vi "AeroQuadUploader32 - Copy.vi"() -> ()   [LabVIEW 2010]
panel:
  in  "WebBrowser":refnum<k7>(container)
  in  "URL":string="http://aq32.aeroquad.com"
  in  "Com Port":refnum<visa-resource-name>
  out "Status":string="AeroQuad 32 Uploader"
  in  "Restart":bool
  in  "Done":bool
  in  "Upload":bool
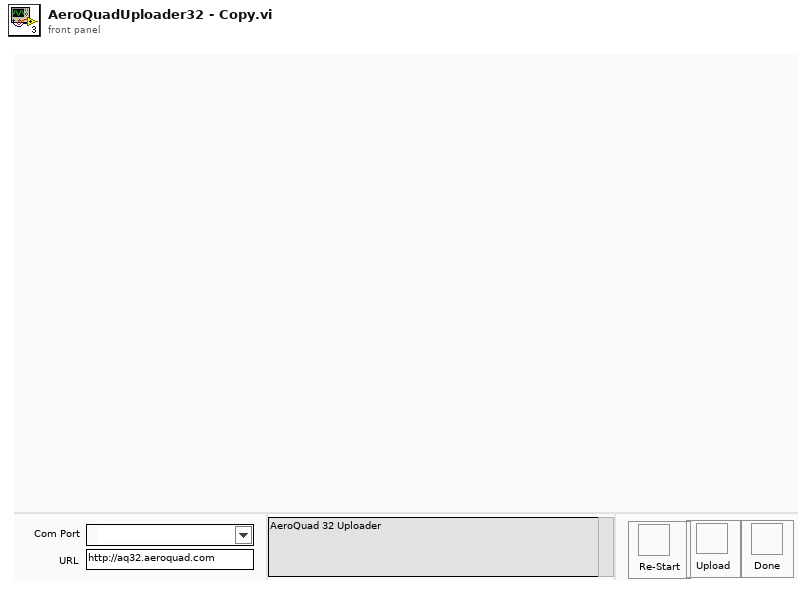
[diagram p1: front panel]
types:
  T1 = cluster{"Connected":bool, "WebBrowser":refnum<k7>, "WorkingFolder":path, "HTML":string}
  T2 = enum16{"Read", "Write", "ReadWrite", "BufferedRead", "BufferedReadWrite"}
  T3 = enum32{"invalid app kind", "Development System", "Run Time System", "Student Edition", "Embedded LabVIEW", "Evaluation", "Custom"}
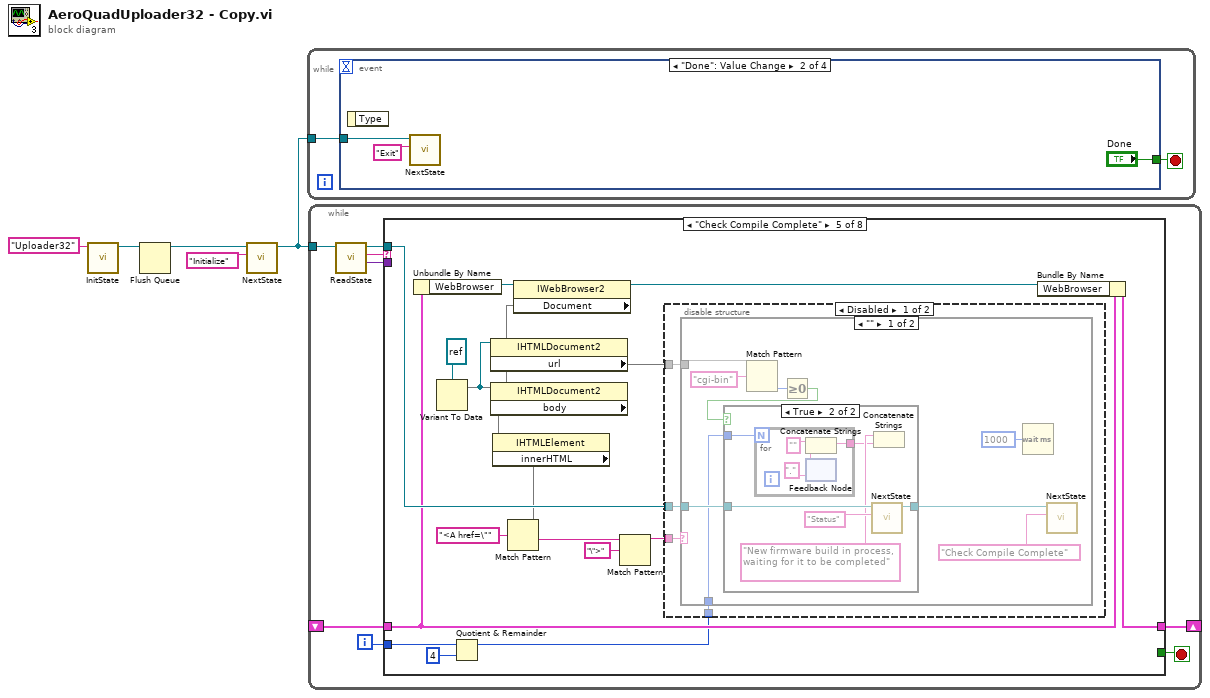
[diagram p0: block diagram]
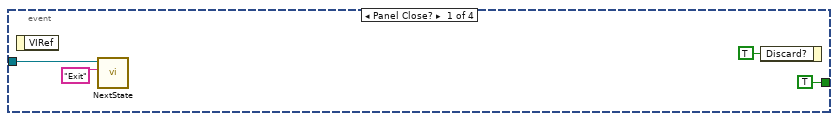
[diagram p2: hidden frame]
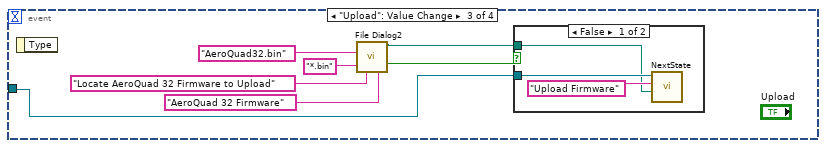
[diagram p3: hidden frame]
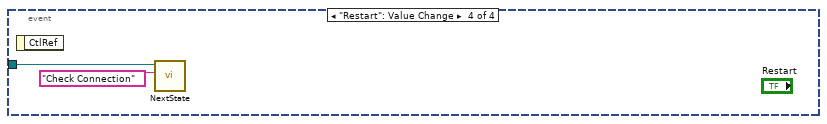
[diagram p5: hidden frame]
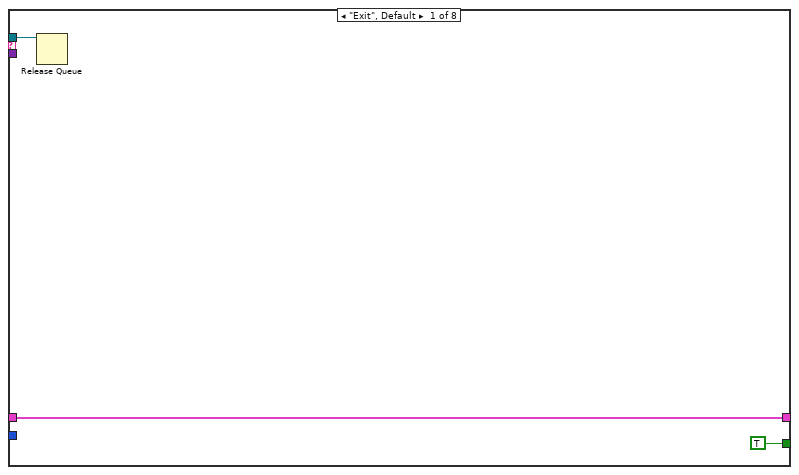
[diagram p6: hidden frame]
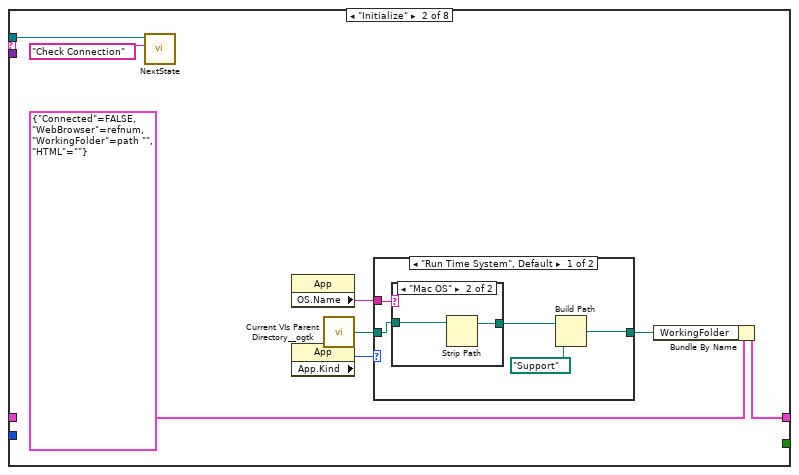
[diagram p7: hidden frame]
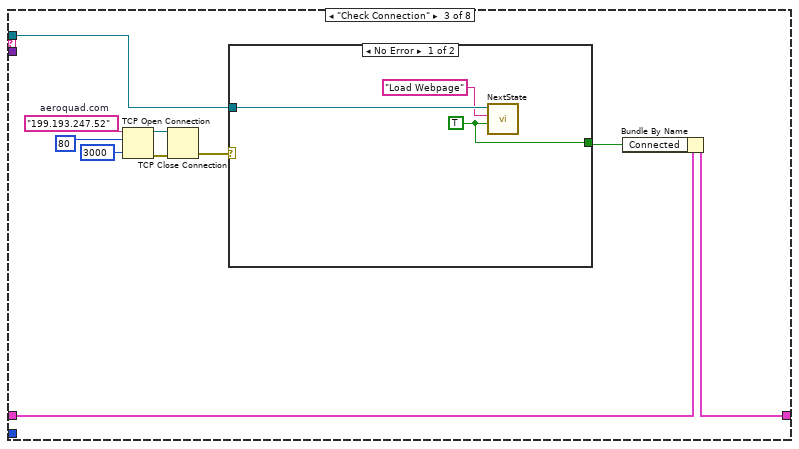
[diagram p10: hidden frame]
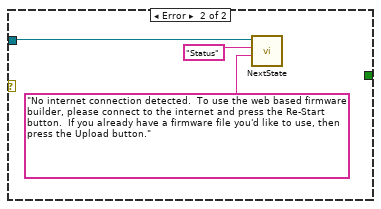
[diagram p11: hidden frame]
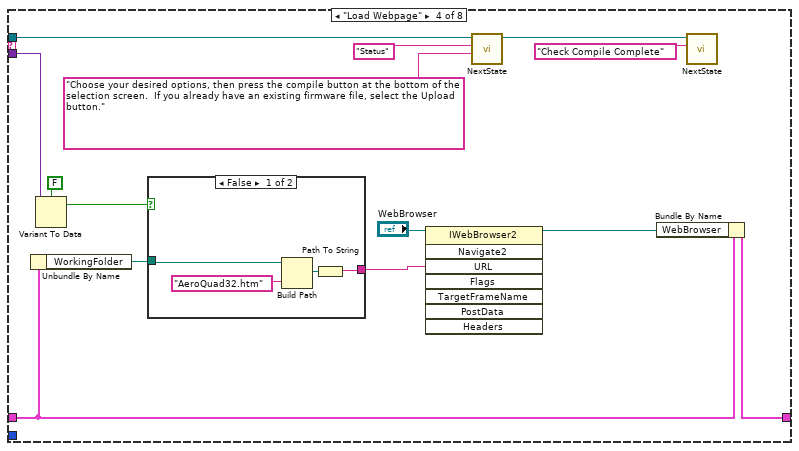
[diagram p12: hidden frame]
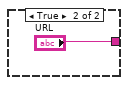
[diagram p13: hidden frame]
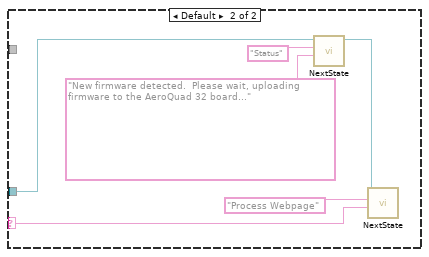
[diagram p15: hidden frame]
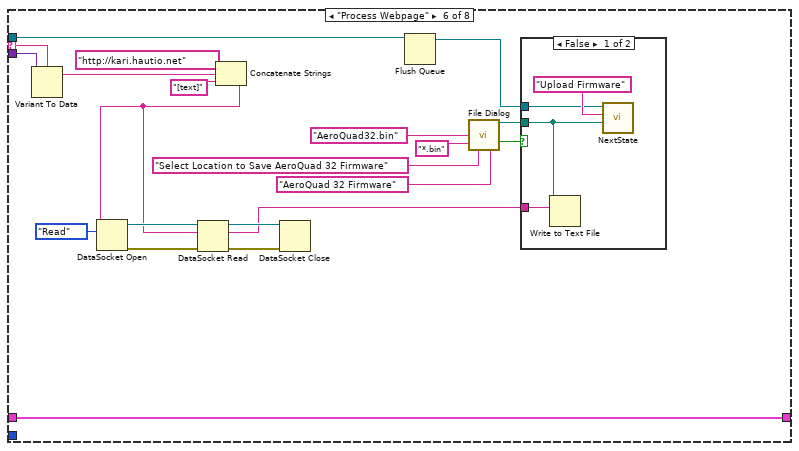
[diagram p17: hidden frame]
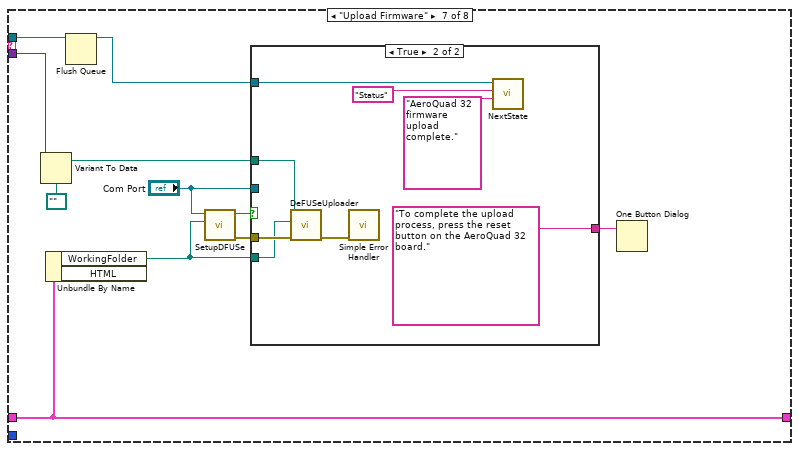
[diagram p19: hidden frame]
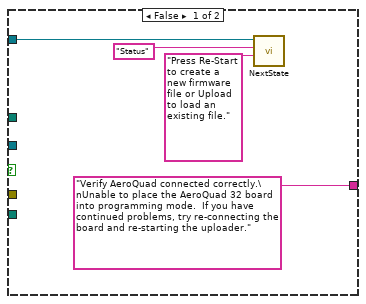
[diagram p20: hidden frame]
diagram:
  n1 = call "InitState.vi"("Name"="Uploader32") -> ("Queue Out"=w1:refnum<queue>)  [unwired: 8 in, 1 out]
  n2 = Flush Queue(queue=w1) -> (queue out=w2:refnum<queue>)  [unwired: 1 in, 2 out]
  n3 = call "NextState.vi"("State"="Initialize", "Queue In"=w2) -> ("Queue Out"=w3:refnum<queue>)  [unwired: 8 in, 1 out]
  n4 = while {
    tunnel: w3 -> [w6]
    stop <- w7 stop-if-true
    n5 = event shown="[1] \"Done\": Value Change" {
      selector: _ -> [_ _ _ _]
      dyn-events: _ -> [_ _ _ _]
      timeout: _ -> [_ _ _ _]
      tunnel: [TRUE ("Done") "Done" _ _] -> w7
      tunnel: w6 -> [w9 w13 w17 w25]
      event Panel Close? {
        n6 = event-data() -> ()  [unwired: 1 in, 1 out]
        n7 = call "NextState.vi"("State"="Exit", "Queue In"=w9) -> ()  [unwired: 8 in, 2 out]
        n8 = event-data("Discard?"=TRUE) -> ()  [unwired: 1 in, 1 out]
      }
      event "Done": Value Change {
        n9 = event-data() -> ()  [unwired: 1 in, 1 out]
        n10 = call "NextState.vi"("State"="Exit", "Queue In"=w13) -> ()  [unwired: 8 in, 2 out]
      }
      event "Upload": Value Change {
        n11 = event-data() -> ()  [unwired: 1 in, 1 out]
        n12 = call "File Dialog2"("prompt"="Locate AeroQuad 32 Firmware to Upload", "default name"="AeroQuad32.bin", "pattern (all files)"="*.bin", "pattern label"="AeroQuad 32 Firmware") -> ("selected path"=w15:path, "cancelled"=w16:bool)  [unwired: 8 in, 2 out]
        n13 = case shown="False" w16 {
          tunnel: w17 -> [w23 _]
          tunnel: w15 -> [w22 _]
          frame False {
            n14 = call "NextState.vi"("Data"=w22, "State"="Upload Firmware", "Queue In"=w23) -> ()  [unwired: 7 in, 2 out]
          }
          frame True {
          }
        }
      }
      event "Restart": Value Change {
        n15 = event-data() -> ()  [unwired: 1 in, 1 out]
        n16 = call "NextState.vi"("State"="Check Connection", "Queue In"=w25) -> ()  [unwired: 8 in, 2 out]
      }
    }
  }
  n17 = while {
    tunnel: w3 -> [w34]
    shift-right: [w29] -> _
    shift-left: _ -> [w28]
    i -> [w27]
    stop <- w30 stop-if-true
    n18 = call "ReadState.vi"("Queue In"=w34) -> ("Data"=w32:variant, "State"=w33:string, "Queue Out"=w31:refnum<queue>)  [unwired: 7 in, 1 out]
    n19 = case shown="\"Check Compile Complete\"" w33 {
      selector: w33 -> [_ _ _ _ _ w157 _ w188]
      tunnel: w32 -> [_ _ _ w84 _ w158 w169 w189]
      tunnel: w31 -> [w35 w45 w57 w74 w107 w154 w164 _]
      tunnel: [TRUE _ _ _ _ _ _ _] -> w30
      tunnel: [w36 w39 w58 w80 w100 w153 w173 w186] -> w29
      tunnel: w28 -> [w36 _ w59 w78 w101 w153 w173 w186]
      tunnel: w27 -> [_ _ _ _ w92 _ _ _]
      frame "Exit", Default {
        n20 = Release Queue(queue=w35) -> ()  [unwired: 2 in, 3 out]
      }
      frame "Initialize" {
        n21 = call "NextState.vi"("State"="Check Connection", "Queue In"=w45) -> ()  [unwired: 8 in, 2 out]
        n22 = property class="App"() -> ("OS.Name"=w41:string)  [unwired: 2 in, 2 out]
        n23 = property class="App"() -> ("App.Kind"=w43:T3)  [unwired: 2 in, 2 out]
        n24 = call <userlib>:"Current VIs Parent Directory__ogtk.vi"() -> ("Parent Directory (+ Relative)"=w42:path)  [unwired: 5 in]
        n25 = case shown="\"Run Time System\", Default" w43 {
          tunnel: [w46 w54] -> w38
          tunnel: w42 -> [w49 w54]
          tunnel: w41 -> [w47 _]
          frame "Run Time System", Default {
            n26 = case shown="\"Mac OS\"" w47 {
              tunnel: [w51 w53] -> w50
              tunnel: w49 -> [w51 w52]
              frame Default {
              }
              frame "Mac OS" {
                n27 = Strip Path(path=w52) -> (stripped path=w53:path)  [unwired: 1 out]
              }
            }
            n28 = Build Path(base path=w50, name or relative path=path "Support") -> (appended path=w46:path)
          }
          frame "Development System" {
          }
        }
        n29 = Bundle By Name(cluster=T1 {"Connected"=FALSE, "WebBrowser"=refnum, "WorkingFolder"=path "", "HTML"=""}, "WorkingFolder"=w38) -> (w39:T1)
      }
      frame "Check Connection" {
        w64 = "199.193.247.52"  # aeroquad.com
        n30 = TCP Open Connection(address=w64, remote port or service name=u16 80, timeout ms (60000)=3000) -> (connection ID=w60:refnum<k5>, error out=w61:errorcluster)  [unwired: 2 in]
        n31 = TCP Close Connection(connection ID=w60, error in (no error)=w61) -> (error out=w55:errorcluster)  [unwired: 1 in, 1 out]
        n32 = case shown="No Error" w55 {
          tunnel: w57 -> [w67 w70]
          tunnel: [w65 _] -> w56
          frame No Error {
            w65 = TRUE
            n33 = call "NextState.vi"("Data"=w65, "State"="Load Webpage", "Queue In"=w67) -> ()  [unwired: 7 in, 2 out]
          }
          frame Error {
            n34 = call "NextState.vi"("Data"="No internet connection detected.  To use the web based firmware builder, please connect to the internet and press the Re-Start button.  If you already have a firmware file you'd like to use, then press the Upload button." ("State"), "State"="Status", "Queue In"=w70) -> ()  [unwired: 7 in, 2 out]
          }
        }
        n35 = Bundle By Name(cluster=w59, "Connected"=w56) -> (w58:T1)
      }
      frame "Load Webpage" {
        n36 = Unbundle By Name(w78) -> ("WorkingFolder"=w77:path)
        n37 = Variant To Data(Variant=w84, type=FALSE) -> (data=w82:bool)  [unwired: 1 in, 1 out]
        n38 = case shown="False" w82 {
          tunnel: [w85 "URL"] -> w81
          tunnel: w77 -> [w86 _]
          frame False {
            n39 = Build Path(base path=w86, name or relative path="AeroQuad32.htm") -> (appended path=w88:path)
            n40 = Path To String(path=w88) -> (string=w85:string)
          }
          frame True {
          }
        }
        n41 = invoke class="IWebBrowser2" method="Navigate2"(reference="WebBrowser", "URL"=w81) -> (reference out=w79:refnum<k7>)  [unwired: 6 in, 7 out]
        n42 = call "NextState.vi"("Data"="Choose your desired options, then press the compile button at the bottom of the selection screen.  If you already have an existing firmware file, select the Upload button." ("State"), "State"="Status", "Queue In"=w74) -> ("Queue Out"=w73:refnum<queue>)  [unwired: 7 in, 1 out]
        n43 = Bundle By Name(cluster=w78, "WebBrowser"=w79) -> (w80:T1)
        n44 = call "NextState.vi"("State"="Check Compile Complete", "Queue In"=w73) -> ()  [unwired: 8 in, 2 out]
      }
      frame "Check Compile Complete" {
        n45 = Unbundle By Name(w101) -> ("WebBrowser"=w105:refnum<k7>)
        n46 = Quotient & Remainder(x=w92, y=4) -> (x-y*floor(x/y)=w90:i32)  [unwired: 1 out]
        n47 = property class="IWebBrowser2"(reference=w105) -> (reference out=w102:refnum<k7>, "Document"=w104)  [unwired: 1 in, 1 out]
        n48 = Variant To Data(Variant=w104, type=refnum<k7> refnum ("WebBrowser")) -> (data=w94:refnum<k7>)  [unwired: 1 in, 1 out]
        n49 = property class="IHTMLDocument2"(reference=w94) -> ("url"=w93)  [unwired: 1 in, 2 out]
        n50 = property class="IHTMLDocument2"(reference=w94) -> ("body"=w103)  [unwired: 1 in, 2 out]
        n51 = property class="IHTMLElement"(reference=w103) -> ("innerHTML"=w98)  [unwired: 1 in, 2 out]
        n52 = Match Pattern(string=w98, regular expression="<A href=\"") -> (after substring=w97:string)  [unwired: 1 in, 3 out]
        n53 = Match Pattern(string=w97, regular expression="\">") -> (before substring=w95:string)  [unwired: 1 in, 3 out]
        n54 = disable-structure shown="Disabled" {
          disable-tunnel: w107 -> [w111 _]
          disable-tunnel: w95 -> [w110 _]
          disable-tunnel: w93 -> [w109 _]
          disable-tunnel: w90 -> [w108 _]
          frame Disabled {
            n55 = case shown="\"\"" w110 {
              selector: w110 -> [_ w136]
              tunnel: w111 -> [w113 w135]
              tunnel: w109 -> [w118 _]
              tunnel: w108 -> [w112 _]
              frame "" {
                n56 = Match Pattern(string=w118, regular expression="cgi-bin") -> (offset past match=w116:i32)  [unwired: 1 in, 3 out]
                n57 = Greater Or Equal To 0?(x=w116) -> (x >= 0?=w115:bool)
                n58 = case shown="True" w115 {
                  tunnel: [w121 w127] -> w114
                  tunnel: w113 -> [w121 w126]
                  tunnel: w112 -> [_ w123]
                  frame False {
                  }
                  frame True {
                    n59 = for {
                      N: w123 -> [_]
                      tunnel: [w128] -> w122
                      n60 = feedback #1(".") -> (w129:string)
                      n61 = Concatenate Strings("", w129) -> (w128:string)
                      n62 = feedback-in #1() -> ()  [unwired: 1 out]
                    }
                    n63 = call "NextState.vi"("State"="Status", "Queue In"=w126) -> ("Queue Out"=w127:refnum<queue>)  [unwired: 8 in, 1 out]
                    n64 = Concatenate Strings("New firmware build in process, waiting for it to be completed" ("State"), w122) -> ()  [unwired: 1 out]
                  }
                }
                n65 = Wait (ms)(milliseconds to wait=u32 1000) -> ()  [unwired: 1 out]
                n66 = call "NextState.vi"("State"="Check Compile Complete", "Queue In"=w114) -> ()  [unwired: 8 in, 2 out]
              }
              frame Default {
                n67 = call "NextState.vi"("Data"="New firmware detected.  Please wait, uploading firmware to the AeroQuad 32 board..." ("State"), "State"="Status", "Queue In"=w135) -> ("Queue Out"=w134:refnum<queue>)  [unwired: 7 in, 1 out]
                n68 = call "NextState.vi"("Data"=w136, "State"="Process Webpage", "Queue In"=w134) -> ()  [unwired: 7 in, 2 out]
              }
            }
          }
          frame Enabled {
          }
        }
        n69 = Bundle By Name(cluster=w101, "WebBrowser"=w102) -> (w100:T1)
      }
      frame "Process Webpage" {
        n70 = Variant To Data(Variant=w158, type=w157) -> (data=w156:string)  [unwired: 1 in, 1 out]
        n71 = Concatenate Strings("http://kari.hautio.net" ("string"), w156, "[text]" ("string")) -> (w140:string)
        n72 = DataSocket Open(10:T2."Read" ("mode"), 11:w140) -> (0:w143:errorcluster, 3:w145:refnum<k13>)  [unwired: 2 in]
        n73 = DataSocket Read(8:w143, 10:w140, 11:w145) -> (0:w142:errorcluster, 2:w139:string, 3:w144:refnum<k13>)  [unwired: 2 in, 4 out]
        n74 = DataSocket Close(8:w142, 11:w144) -> ()  [unwired: 1 in, 2 out]
        n75 = Flush Queue(queue=w154) -> (queue out=w138:refnum<queue>)  [unwired: 1 in, 2 out]
        n76 = call "File Dialog"("prompt"="Select Location to Save AeroQuad 32 Firmware", "default name"="AeroQuad32.bin", "pattern (all files)"="*.bin", "pattern label"="AeroQuad 32 Firmware") -> ("selected path"=w151:path, "cancelled"=w152:bool)  [unwired: 8 in, 2 out]
        n77 = case shown="False" w152 {
          tunnel: w139 -> [w162 _]
          tunnel: w151 -> [w159 _]
          tunnel: w138 -> [w160 _]
          frame False {
            n78 = Write to Text File(file (use dialog)=w159, text=w162) -> ()  [unwired: 2 in, 3 out]
            n79 = call "NextState.vi"("Data"=w159, "State"="Upload Firmware", "Queue In"=w160) -> ()  [unwired: 7 in, 2 out]
          }
          frame True {
          }
        }
      }
      frame "Upload Firmware" {
        n80 = Variant To Data(Variant=w169, type=path "") -> (data=w167:path)  [unwired: 1 in, 1 out]
        n81 = Unbundle By Name(w173) -> ("WorkingFolder"=w166:path)  [unwired: 1 out]
        n82 = Flush Queue(queue=w164) -> (queue out=w163:refnum<queue>)  [unwired: 1 in, 2 out]
        n83 = call "SetupDFUSe.vi"("Working Directory"=w166, "Serial Port"="Com Port") -> ("Error"=w170:errorcluster, "Success"=w172:bool)  [unwired: 7 in]
        n84 = case shown="True" w172 {
          tunnel: "Com Port" -> [_ _]
          tunnel: w170 -> [_ w185]
          tunnel: w167 -> [_ w183]
          tunnel: w166 -> [_ w182]
          tunnel: ["Verify AeroQuad connected correctly.\nUnable to place the AeroQuad 32 board into programming mode.  If you have continued problems, try re-connecting the board and re-starting the uploader." ("message") "To complete the upload process, press the reset button on the AeroQuad 32 board." ("message")] -> w165
          tunnel: w163 -> [w174 w178]
          frame False {
            n85 = call "NextState.vi"("Data"="Press Re-Start to create a new firmware file or Upload to load an existing file." ("State"), "State"="Status", "Queue In"=w174) -> ()  [unwired: 7 in, 2 out]
          }
          frame True {
            n86 = call "DeFUSeUploader.vi"("Error In"=w185, "DFU-Util Working Directory"=w182, "Binary Filename"=w183) -> ("Error Out"=w184:errorcluster)  [unwired: 8 in]
            n87 = call <vilib>:"Simple Error Handler.vi"("error in (no error)"=w184) -> ()  [unwired: 4 in, 5 out]
            n88 = call "NextState.vi"("Data"="AeroQuad 32 firmware upload complete." ("State"), "State"="Status", "Queue In"=w178) -> ()  [unwired: 7 in, 2 out]
          }
        }
        n89 = One Button Dialog(message=w165) -> ()  [unwired: 1 in, 1 out]
      }
      frame "Status" {
        n90 = Variant To Data(Variant=w189, type=w188) -> (data=→"Status":string)  [unwired: 1 in, 1 out]
      }
    }
  }
